vi "NewConfig.vi"(8 "error in (no error)":errorcluster, 11 "xceRootNode in":refnum<class "xceRootNode.lvclass">) -> (0 "error out":errorcluster, 1 "cancelled":bool, 3 "xceRootNode out":refnum<class "xceRootNode.lvclass">)   [LabVIEW 2013, in "xceRootNode.lvclass"]
doc: "Starts a new configuration. Prompts the user if they would like to save the current configuration before starting a new one."
uses:
  xceRootNode.lvclass
  xceRootNode.lvclass/xceRootNode.ctl
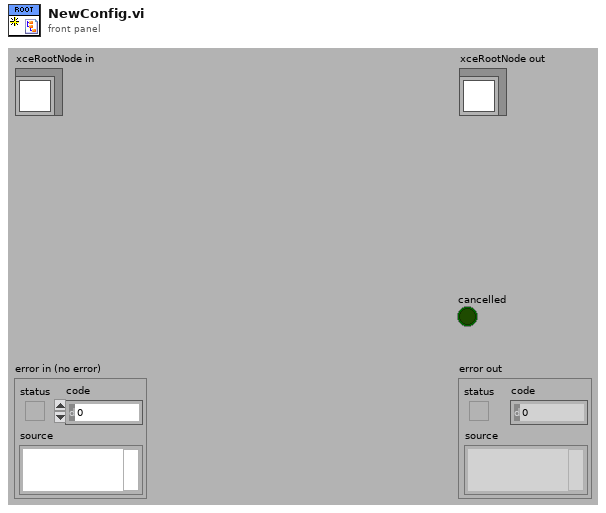
[diagram p1: front panel]
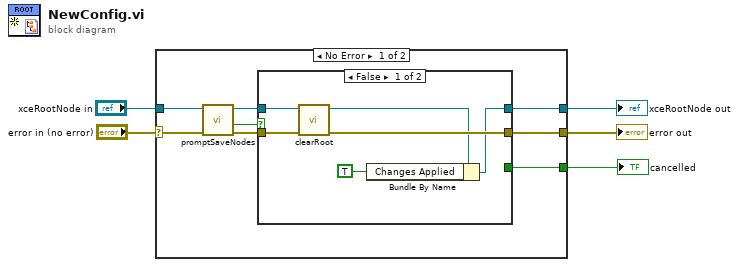
[diagram p0: block diagram]
diagram:
  n1 = case shown="No Error" "error in (no error)" {
    selector: "error in (no error)" -> [w12 w24]
    tunnel: [w7 w24] -> w4
    tunnel: [w8 w23] -> w2
    tunnel: "xceRootNode in" -> [w13 w23]
    tunnel: [w6 _] -> w1
    frame No Error {
      n2 = call "promptSaveNodes.vi"("error in (no error)"=w12, "xceRootNode in"=w13) -> ("error out"=w10:errorcluster, "cancelled"=w11:bool, "xceRootNode out"=w9:refnum<class "xceRootNode.lvclass">)  [unwired: 7 in]
      n3 = case shown="False" w11 {
        selector: w11 -> [_ w20]
        tunnel: w10 -> [w18 w21]
        tunnel: w9 -> [w19 w22]
        tunnel: [w14 w22] -> w8
        tunnel: [w17 w21] -> w7
        tunnel: [_ w20] -> w6
        frame False {
          n4 = call "clearRoot.vi"("error in (no error)"=w18, "xceRootNode in"=w19) -> ("error out"=w17:errorcluster, "xceRootNode out"=w15:refnum<class "xceRootNode.lvclass">)  [unwired: 8 in]
          n5 = Bundle By Name(cluster=w15, "Changes Applied"=TRUE) -> (w14:refnum<class "xceRootNode.lvclass">)
        }
        frame True {
        }
      }
    }
    frame Error {
    }
  }
  "error out" <- w4
  "xceRootNode out" <- w2
  "cancelled" <- w1
